vi "Wait for WLM Event.vi"(8 "error in (no error)":errorcluster, 9 "Callback/Wait Mode":i16(ring)=42 items=["cmiTemperature"=14, "cmiWavelength1"=42, "cmiWavelength2"=43, "cmiWavelength3"=90, "cmiWavelength4"=91, "cmiWavelength5"=92, "cmiWavelength6"=93, "cmiWavelength7"=94, "cmiWavelength8"=95, "cmiLinewidth"=44, "cmiDistance"=69, "cmiAnalogIn"=66, "cmiAnalogOut"=67, "cmiExposureMode"=6, "cmiResultMode"=1, "cmiRange"=2, "cmiPulseMode"=3, "cmiWideMode"=4, "cmiFastMode"=5, "cmiDisplayMode"=17, "cmiAnalysisMode"=32, "cmiReduced"=12, "cmiLink"=15, "cmiOperation"=16, "cmiVersion0"=31, "cmiVersion1"=96, "cmiDLLDetach"=30, "cmiDLLAttach"=121, "cmiMin1"=22, "cmiMin2"=24, "cmiMax1"=23, "cmiMax2"=25, "cmiExposureValue11"=7, "cmiExposureValue12"=125, "cmiExposureValue13"=126, "cmiExposureValue14"=127, "cmiExposureValue15"=128, "cmiExposureValue16"=129, "cmiExposureValue17"=130, "cmiExposureValue18"=131, "cmiExposureValue21"=8, "cmiExposureValue22"=132, "cmiExposureValue23"=133, "cmiExposureValue24"=134, "cmiExposureValue25"=135, "cmiExposureValue26"=136, "cmiExposureValue27"=137, "cmiExposureValue28"=138], 10 "device serial #":i32) -> (0 "error out":errorcluster, 1 "Wait Return Values":T1 items=["unknown event or error"=-2, "timeout"=-1, "mechanism not installed"=0, "change + other results"=1, "change: no other results"=2], 2 "return value":i32)   [LabVIEW 2009, in "HighFinesse WS5.lvlib"]
doc: "Waits for the given event, and then returns the reason it returned. It may return with one of the following results: (a) it receive measurement or state-change information and there are still other results; (b) same as (a), but there are no additional results; (c) no wait event is currently installed; (d) timeout; (e) an unknown event or error occurred. These last three are considered errors.\n\n<B>Note: Before this can be used, a wait event must be installed; see Wait Event.vi</B>."
uses:
  HighFinesse WS5.lvlib
  Control typedefs.llb/Wait Return Values.ctl
  <vilib>/Utility/error.llb/DialogType.ctl
  Program Files/HighFinesse/Wavelength Meter WS5 399/Com-Test/wlmData.dll
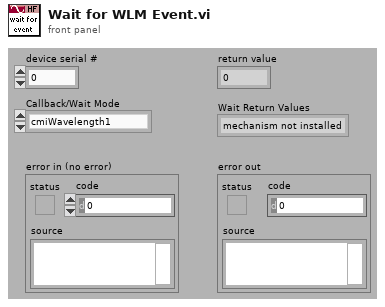
[diagram p1: front panel]
types:
  T1 = typedef "HighFinesse WS5.lvlib/Wait Return Values.ctl" = i32
  T2 = typedef "DialogType.ctl" = u16
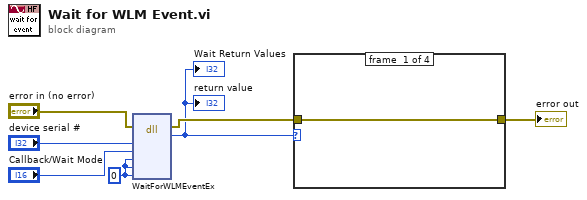
[diagram p0: block diagram]
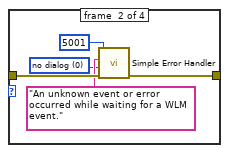
[diagram p2: hidden frame]
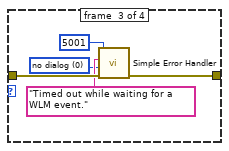
[diagram p3: hidden frame]
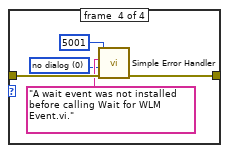
[diagram p4: hidden frame]
diagram:
  w2 = 0 ("Res1")
  n1 = dll-call lib="C:/Program Files/HighFinesse/Wavelength Meter WS5 399/Com-Test/wlmData.dll" fn="WaitForWLMEventEx"(error in="error in (no error)", "Ver"="device serial #", "Mode"="Callback/Wait Mode", "IntVal"=w2, "DblVal"=w2, "Res1"=w2) -> (error out=w6:errorcluster, "return type"=w1:i32)  [unwired: 5 in, 3 out]
  "return value" <- w1
  "Wait Return Values" <- w1
  n2 = case shown="-1" w1 {
    tunnel: w6 -> [w8 w13 w18 w23]
    tunnel: [w8 w10 w15 w20] -> w5
    frame #0 {
    }
    frame #1 {
      w11 = T2 0 items=["no dialog", "OK message", "continue or stop message", "OK message + warnings", "continue/stop + warnings"] ("type of dialog (OK msg:1)")
      n3 = call <vilib>:"Simple Error Handler.vi"("error code (no error:0)"=5001, "error source (\" \")"="An unknown event or error occurred while waiting for a WLM event." ("error source (\" \")"), "type of dialog (OK msg:1)"=w11, "error in (no error)"=w13) -> ("error out"=w10:errorcluster)  [unwired: 5 out]
    }
    frame #2 {
      w16 = T2 0 items=["no dialog", "OK message", "continue or stop message", "OK message + warnings", "continue/stop + warnings"] ("type of dialog (OK msg:1)")
      n4 = call <vilib>:"Simple Error Handler.vi"("error code (no error:0)"=5001, "error source (\" \")"="Timed out while waiting for a WLM event." ("error source (\" \")"), "type of dialog (OK msg:1)"=w16, "error in (no error)"=w18) -> ("error out"=w15:errorcluster)  [unwired: 5 out]
    }
    frame #3 {
      w21 = T2 0 items=["no dialog", "OK message", "continue or stop message", "OK message + warnings", "continue/stop + warnings"] ("type of dialog (OK msg:1)")
      n5 = call <vilib>:"Simple Error Handler.vi"("error code (no error:0)"=5001, "error source (\" \")"="A wait event was not installed before calling Wait for WLM Event.vi." ("error source (\" \")"), "type of dialog (OK msg:1)"=w21, "error in (no error)"=w23) -> ("error out"=w20:errorcluster)  [unwired: 5 out]
    }
  }
  "error out" <- w5
